vi "serial_line_to_array.vi"(11 "input string":string) -> (3 "Array":sgl[](array[numeric]))   [LabVIEW 2018]
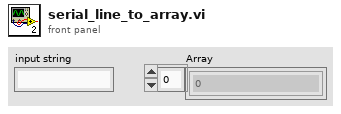
[diagram p1: front panel]
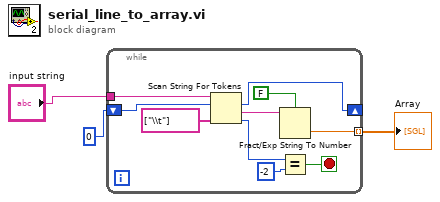
[diagram p0: block diagram]
diagram:
  n1 = while {
    shift-right: [w9] -> _
    shift-left: 0 ("offset past token") -> [w13]
    tunnel: [w5] -> w2 mode=indexing
    tunnel: "input string" -> [w4]
    stop <- w8 stop-if-true
    n2 = Scan String For Tokens(6:string[] ["\\t"] ("delimiters (\\s,\\t,\\r,\\n)"), 8:w13, 9:w4) -> (0:w11:i32, 1:w6:string, 2:w9:i32)  [unwired: 3 in, 1 out]
    n3 = Fract/Exp String To Number(use system decimal point (T)=FALSE, string=w6) -> (number=w5:dbl)  [unwired: 2 in, 1 out]
    n4 = Equal?(x=w11, y=-2) -> (x = y?=w8:bool)
  }
  "Array" <- w2
